vi "subDFD_Cascade Multirate Filters with Multirate Filter.vi"(8 "error in (no error)":errorcluster, 10 "multirate filters":T1[](array[typedef]) {"mMRate_SumWl" min=1 max=32 step=1; "mMRate_InputIwl" min=1 max=32 step=1; "mMRate_GainWl" min=1 max=32 step=1; "mMRate_OutputWl" min=1 max=32 step=1; "mMRate_InputWl" min=1 max=32 step=1; "mMRate_CoefWl" min=1 max=32 step=1; "mMRate_Mode" items=["Default"=-1, "No Rate Change"=0, "Interpolation"=1, "Decimation"=2, "Interpolated"=3, "Rational"=4]}, 11 "multirate filter":T1 {"mMRate_SumWl" min=1 max=32 step=1; "mMRate_InputIwl" min=1 max=32 step=1; "mMRate_GainWl" min=1 max=32 step=1; "mMRate_OutputWl" min=1 max=32 step=1; "mMRate_InputWl" min=1 max=32 step=1; "mMRate_CoefWl" min=1 max=32 step=1; "mMRate_Mode" items=["Default"=-1, "No Rate Change"=0, "Interpolation"=1, "Decimation"=2, "Interpolated"=3, "Rational"=4]}) -> (0 "error out":errorcluster, 3 "cascaded filters":T1[](array[typedef]) {"mMRate_SumWl" min=1 max=32 step=1; "mMRate_InputIwl" min=1 max=32 step=1; "mMRate_GainWl" min=1 max=32 step=1; "mMRate_OutputWl" min=1 max=32 step=1; "mMRate_InputWl" min=1 max=32 step=1; "mMRate_CoefWl" min=1 max=32 step=1; "mMRate_Mode" items=["Default"=-1, "No Rate Change"=0, "Interpolation"=1, "Decimation"=2, "Interpolated"=3, "Rational"=4]})   [LabVIEW 2023]
uses:
  <vilib>/addons/Digital Filter Design/_Objects.llb/DFD Multirate Filter Obj.ctl
  <vilib>/addons/Digital Filter Design/_Objects.llb/DFD Multirate Mode.ctl
  <vilib>/addons/Digital Filter Design/_Objects.llb/DFD Coef Norm Type.ctl
  <vilib>/addons/Digital Filter Design/_Objects.llb/DFD Round-off Mode.ctl
  <vilib>/addons/Digital Filter Design/_Objects.llb/DFD FXP MRate Multiply Mode.ctl
  <vilib>/addons/Digital Filter Design/_Objects.llb/DFD Multirate Filtering Mode.ctl
  <vilib>/addons/Digital Filter Design/FilterLib.llb/DFD Build MRate Filter from FIR Filter.vi
  <vilib>/addons/Digital Filter Design/NI_DigFilterLicensed.lvlib
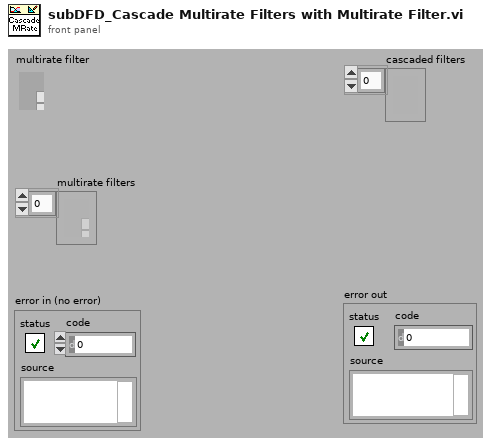
[diagram p1: front panel]
types:
  T1 = typedef "NI_DigFilterLicensed.lvlib/DFD Multirate Filter Obj.ctl" = cluster{"mMRate_Structure":enum16{"CIC", "FIR", "IIR", "Lattice"}, "mMRate_Mode":T2, "mMRate_Factor":i32, "mMRate_FIRParams":cluster{"mMRate_FIR_H":dbl[], "mMRate_FIR_IsNyquist?":bool, "mMRate_FIR_IsSymmetric?":bool}, "mMRate_CICParams":cluster{"mMRate_CIC_#Stage":i32, "mMRate_CIC_Lag":i32, "mMRate_CIC_Type":enum16{"Lowpass", "Highpass"}}, "mMRate_Order":i32, "mMRate_Version":string, "mMRate_Comments":string, "mMRate_RationalFactor":cluster{"mMRate_L":i32, "mMRate_M":i32}, "mMRate_Fs":dbl, "mMRate_Quantized?":bool, "mMRate_QFilterGain":dbl, "mMRate_CoefWl":i16, "mMRate_Scaling":cluster{"mMRate_ScaleByPowerOf2?":bool, "mMRate_ScaleType":T3}, "mMRate_InputWl":i16, "mMRate_OutputWl":i16, "mMRate_OutputMode":T4, "mMRate_MultMode":T5, "mMRate_BitPruning":bool, "mMRate_GainWl":i16, "mMRate_OutputFwl":i16, "mMRate_SumIwl":i16, "mMRate_InputIwl ":i16, "mMRate_SumWl":i16, "mMRate_CoefIwl":i16}
  T2 = typedef "NI_DigFilterLicensed.lvlib/DFD Multirate Mode.ctl" = i16
  T3 = typedef "NI_DigFilterLicensed.lvlib/DFD Coef Norm Type.ctl" = enum16{"No Norm", "Time Domain 1-Norm", "Time Domain 2-Norm", "Time Domain Inf-Norm"}
  T4 = typedef "NI_DigFilterLicensed.lvlib/DFD Round-off Mode.ctl" = enum16{"Nearest", "Truncation"}
  T5 = typedef "NI_DigFilterLicensed.lvlib/DFD FXP MRate Multiply Mode.ctl" = enum16{"Truncated", "Full"}
  T6 = typedef "NI_DigFilterLicensed.lvlib/DFD Multirate Filtering Mode.ctl" = u16
  T7 = typedef "NI_DigFilterLicensed.lvlib/DFD Filter Obj.ctl" = cluster{"mSRate_Fs":dbl, "mSRate_Version":string, "mSRate_Comments":string, "mSRate_OrgCoef":T8, "mSRate_CurCoef":T8, "mSRate_Quantized?":bool, "mSRate_QCoef":T8, "mSRate_QSettings":T10[], "mSRate_Order":i32, "mSRate_Scaling":cluster{"mSRate_ScaleByPowerOf2?":bool, "mSRate_ScaleType":T3}}
  T8 = typedef "NI_DigFilterLicensed.lvlib/DFD Filter Coef.ctl" = cluster{"type":T9, "gain":dbl, "coef a (k)":dbl[], "coef b (v)":dbl[]}
  T9 = typedef "NI_DigFilterLicensed.lvlib/DFD Filter Structure Type Selector.ctl" = enum16{"Undefined", "FIR Direct Form", "FIR Direct Form Transposed", "FIR Symmetric", "FIR Antisymmetric", "IIR Direct Form I", "IIR Direct Form I Transposed", "IIR Direct Form II", "IIR Direct Form II Transposed", "IIR Cascaded Second Order Sections Form I", "IIR Cascaded Second Order Sections Form I Transposed", "IIR Cascaded Second Order Sections Form II", "IIR Cascaded Second Order Sections Form II Transposed", "Lattice Allpass (basic sections)", "Lattice Allpass (one multiplier sections)", "Lattice Allpass (normalized sections)", "Lattice AR (basic sections)", "Lattice AR (one multiplier sections)", "Lattice AR (normalized sections)", "Lattice MA (minimum phase)", "Lattice MA (maximum phase)", "Lattice ARMA (basic sections)", "Lattice ARMA (one multiplier sections)", "Lattice ARMA (normalized sections)"}
  T10 = typedef "NI_DigFilterLicensed.lvlib/dfd_Internal Quantization Settings.ctl" = cluster{"source":T11, "wl":i16, "iwl":i16, "overflow mode":enum16{"Saturation", "Wrap"}, "rounding mode":enum16{"Nearest", "Truncation"}, "signed?":bool}
  T11 = typedef "NI_DigFilterLicensed.lvlib/dfd_Internal Quantization Srcs.ctl" = u16
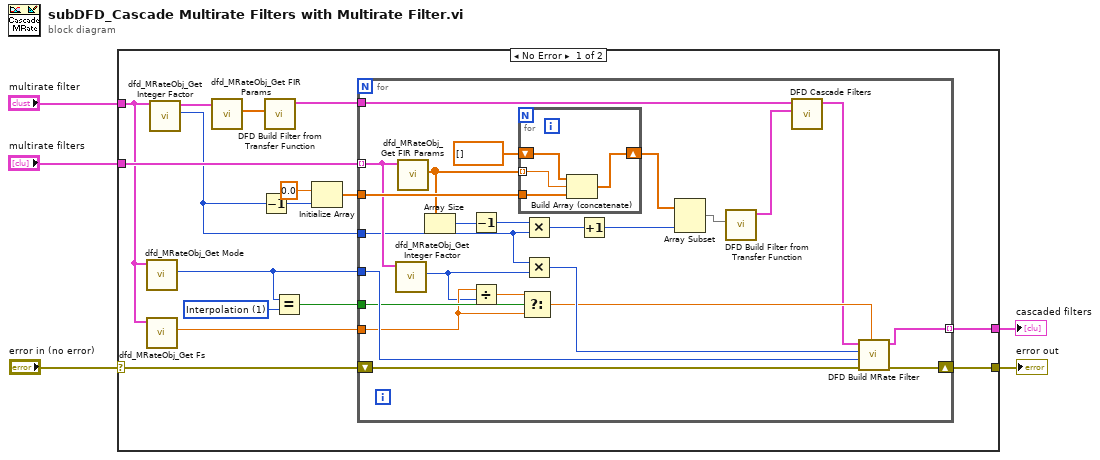
[diagram p0: block diagram]
diagram:
  n1 = case shown="No Error" "error in (no error)" {
    selector: "error in (no error)" -> [w10 w50]
    tunnel: "multirate filters" -> [w21 _]
    tunnel: [w20 _] -> w4
    tunnel: "multirate filter" -> [w6 _]
    tunnel: [w9 w50] -> w1
    frame No Error {
      w15 = T6 1 items=["No Rate Change", "Interpolation", "Decimation"] ("filtering mode")
      n2 = call <vilib>:"dfd_MRateObj_Get Mode.vi"("multirate filter in"=w6) -> ("mode"=w14:T2)  [unwired: 9 in, 1 out]
      n3 = call <vilib>:"dfd_MRateObj_Get Fs.vi"("multirate filter in"=w6) -> ("fs"=w12:dbl)  [unwired: 9 in, 1 out]
      n4 = call <vilib>:"dfd_MRateObj_Get Integer Factor.vi"("multirate filter in"=w6) -> ("factor"=w17:i32, "dup multirate filter"=w11:T1)  [unwired: 9 in]
      n5 = call <vilib>:"dfd_MRateObj_Get FIR Params.vi"("multirate filter in"=w11) -> ("h(n)"=w8:dbl[])  [unwired: 7 in, 3 out]
      n6 = Decrement(x=w17) -> (x-1=w19:i32)
      n7 = call <vilib>:"DFD Build Filter from Transfer Function.vi"("numerator"=w8) -> ("filter out"=w7:T7)  [unwired: 9 in, 1 out]
      n8 = Equal?(x=w14, y=w15) -> (x = y?=w13:bool)
      n9 = Initialize Array(0.0 ("element"), w19) -> (w16:dbl[])
      n10 = for {
        tunnel: w21 -> [w31] mode=indexing
        tunnel: w7 -> [w33]
        tunnel: w17 -> [w27]
        tunnel: w14 -> [w41]
        tunnel: [w43] -> w20 mode=indexing
        tunnel: w16 -> [w42]
        tunnel: w13 -> [w40]
        tunnel: w12 -> [w39]
        shift-right: [w34] -> w9
        shift-left: w10 -> [w35]
        n11 = call <vilib>:"dfd_MRateObj_Get Integer Factor.vi"("multirate filter in"=w31) -> ("factor"=w38:i32)  [unwired: 9 in, 1 out]
        n12 = call <vilib>:"dfd_MRateObj_Get FIR Params.vi"("multirate filter in"=w31) -> ("h(n)"=w30:dbl[])  [unwired: 7 in, 3 out]
        n13 = Array Size(array=w30) -> (size(s)=w28:i32)
        n14 = Decrement(x=w28) -> (x-1=w25:i32)
        n15 = Divide(x=w39, y=w38) -> (x/y=w37:dbl)
        n16 = for {
          tunnel: w30 -> [w47] mode=indexing
          tunnel: w42 -> [w46]
          shift-right: [w48] -> w29
          shift-left: dbl[] [] ("initialized array") -> [w49]
          n17 = Build Array (concatenate)(w49, w47, w46) -> (w48:dbl[])
        }
        n18 = Select(t=w37, s=w40, f=w39) -> (s? t:f=w36:dbl)
        n19 = Multiply(x=w25, y=w27) -> (x*y=w26:i32)
        n20 = Multiply(x=w27, y=w38) -> (x*y=w44:i32)
        n21 = Increment(x=w26) -> (x+1=w24:i32)
        n22 = Array Subset(array=w29, length=w24) -> (w23:dbl[])  [unwired: 1 in]
        n23 = call <vilib>:"DFD Build Filter from Transfer Function.vi"("numerator"=w23) -> ("filter out"=w32:T7)  [unwired: 9 in, 1 out]
        n24 = call <vilib>:"DFD Cascade Filters.vi"("filter in 2"=w32, "filter in 1"=w33) -> ("filter out"=w22:T7)  [unwired: 8 in, 1 out]
        n25 = call-poly <vilib>:"DFD Build MRate Filter.vi"("fs in [Hz]"=w36, "error in (no error)"=w35, "filtering mode"=w41, "factor"=w44, "filter in"=w22) -> ("error out"=w34:errorcluster, "multirate filter out"=w43:T1)  [unwired: 5 out]
      }
    }
    frame Error {
    }
  }
  "cascaded filters" <- w4
  "error out" <- w1
